vi "Array1.vi"() -> ()   [LabVIEW 2017]
uses:
  <vilib>/Analysis/Matrix/Datatypes/RealMatrix.ctl
  <vilib>/Analysis/Matrix/Numeric/Multiply/Multiply - RM,RM.vi
  <vilib>/Analysis/Matrix/NI_Matrix.lvlib
panel:
  out "M1 x M2":T1
  in  "Matrix 2":T1
  in  "Variable8":dbl[](array[numeric])
  in  "Variable7":dbl[](array[numeric])
  in  "Variable6":dbl[](array[numeric])
  in  "Variable5":dbl[](array[numeric])
  in  "Variable4":dbl[](array[numeric])
  in  "Variable3":dbl[](array[numeric])
  in  "Variable2":dbl[](array[numeric])
  in  "Variable1":dbl[](array[numeric])
  out "Matrix 1":T1
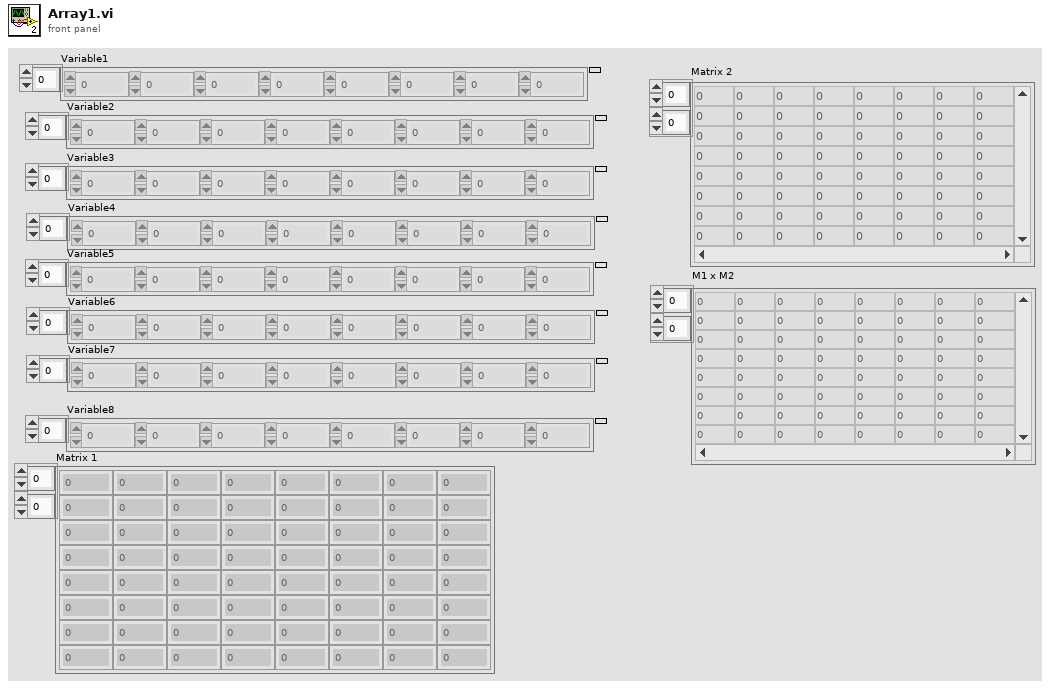
[diagram p1: front panel]
types:
  T1 = typedef "NI_Matrix.lvlib/RealMatrix.ctl" = dbl[][]
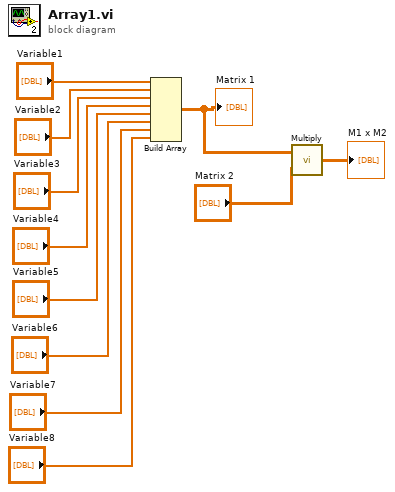
[diagram p0: block diagram]
diagram:
  n1 = Build Array("Variable1", "Variable2", "Variable3", "Variable4", "Variable5", "Variable6", "Variable7", "Variable8") -> (w2:T1)
  "Matrix 1" <- w2
  n2 = call-poly <vilib>:"Multiply.vi"("Real Matrix B"="Matrix 2", "Real Matrix A"=w2) -> ("A * B"=→"M1 x M2":T1)
